vi "WPI_DashboardSD Updates.vi"(10 "Operation":enum16{"Append", "Read and Clear"}(ring)=enum."Read and Clear", 11 "Updates":T5) -> (3 "Collected Data":T6(array[cluster]))   [LabVIEW 2017]
uses:
  <vilib>/Rock Robotics/Network Tables/Protocol Operations.ctl
  <vilib>/Rock Robotics/Network Tables/Field Data.ctl
  <vilib>/Rock Robotics/Network Tables/Field Type.ctl
  <vilib>/Rock Robotics/Network Tables/Sequence.ctl
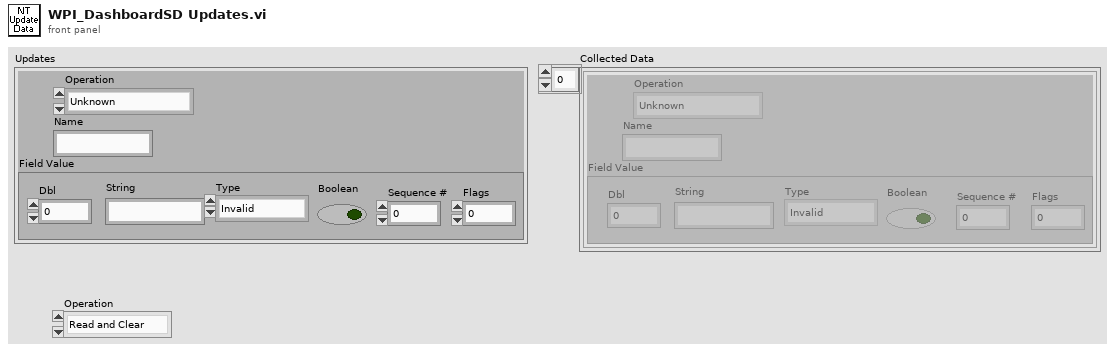
[diagram p1: front panel]
types:
  T1 = typedef "Protocol Operations.ctl" = enum16{"Unknown", "Keep Alive", "Client Hello", "Version not supported", "Server Hello Complete", "Assign", "Update", "No Op", "Server Hello", "Client Hello Complete", "Update Flags", "Delete Entry", "Delete All", "RPC Exec", "RPC Response"}
  T2 = typedef "Field Data.ctl" = cluster{"Dbl":dbl, "String":string, "Type":T3, "Boolean":bool, "Sequence #":T4, "Flags":u8}
  T3 = typedef "Field Type.ctl" = enum8{"Invalid", "Bool", "Numeric", "String", "Raw", "Boolean Array", "Numeric Array", "String Array", "RPC"}
  T4 = typedef "Sequence.ctl" = u16
  T5 = cluster{"Operation":T1, "Name":string, "Field Value":T2}
  T6 = cluster{"Operation":T1, "Name":string, "Field Value":T2}[]
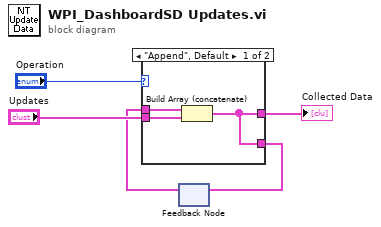
[diagram p0: block diagram]
diagram:
  n1 = feedback #1() -> (w1:T6)  [unwired: 1 in]
  n2 = case shown="\"Append\", Default" "Operation" {
    tunnel: [w7 w9] -> w5
    tunnel: "Updates" -> [w8 _]
    tunnel: [w7 _] -> w2
    tunnel: w1 -> [w6 w9]
    frame "Append", Default {
      n3 = Build Array (concatenate)(w6, w8) -> (w7:T6)
    }
    frame "Read and Clear" {
    }
  }
  "Collected Data" <- w5
  n4 = feedback-in #1(w2) -> ()
